vi "Log Writer.vi"(8 "error in (no error)":errorcluster) -> (0 "error out":errorcluster)   [LabVIEW 2026, in "PXI_Common.lvlib"]
uses:
  PXI_Common.lvlib
  Types/Typedef/Log Message Levels.ctl
  Types/Enum/Bench Modules.ctl
  Types/Typedef/Log Message.ctl
panel:
  out "date/time string":string
  in  "Log Table":string[][](table)
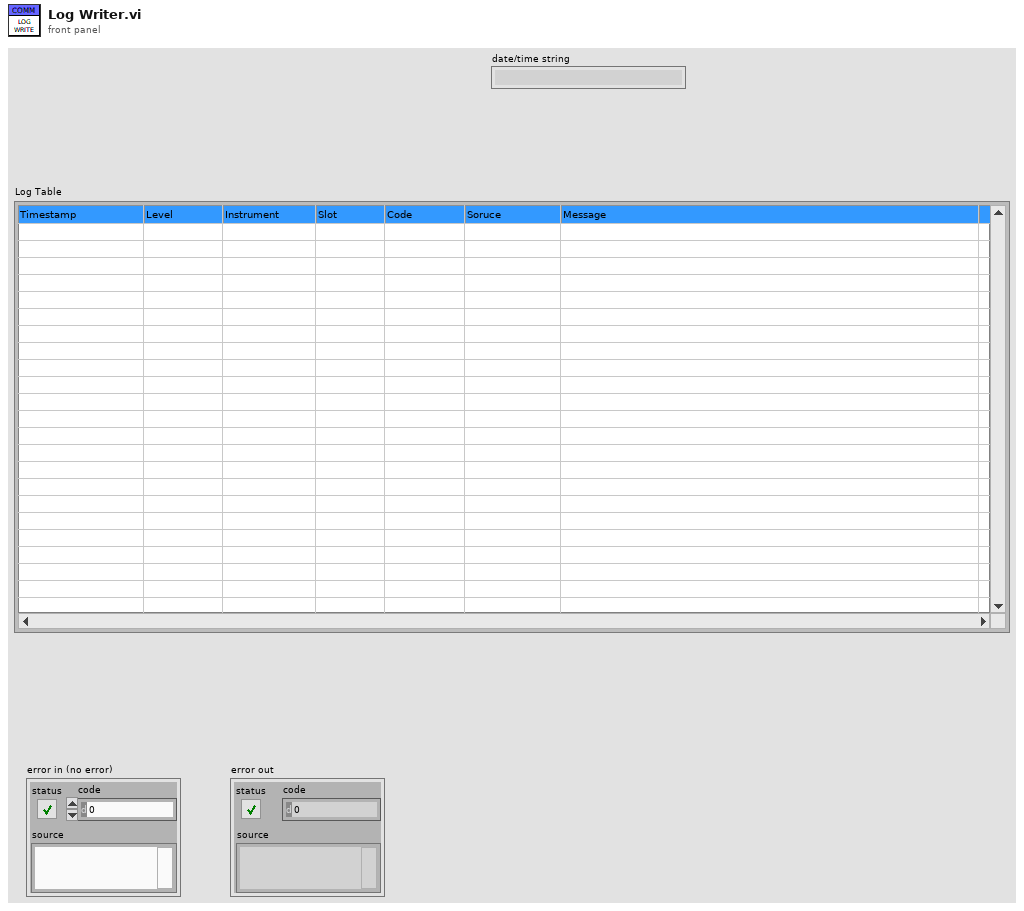
[diagram p1: front panel]
types:
  T1 = typedef "PXI_Common.lvlib/Log Message.ctl" = cluster{"Timestamp":string, "Level":T2, "Instrument":T3, "Slot":string, "Code":i32, "Soruce":string, "Message":string}
  T2 = typedef "PXI_Common.lvlib/Log Message Levels.ctl" = enum16{"DEBUG", "INFO", "WARNING", "ERROR"}
  T3 = typedef "PXI_Common.lvlib/Bench Modules.ctl" = enum16{"Common", "PXI4072", "PXI6259", "PXI6224", "PXI4130", "PXI8431"}
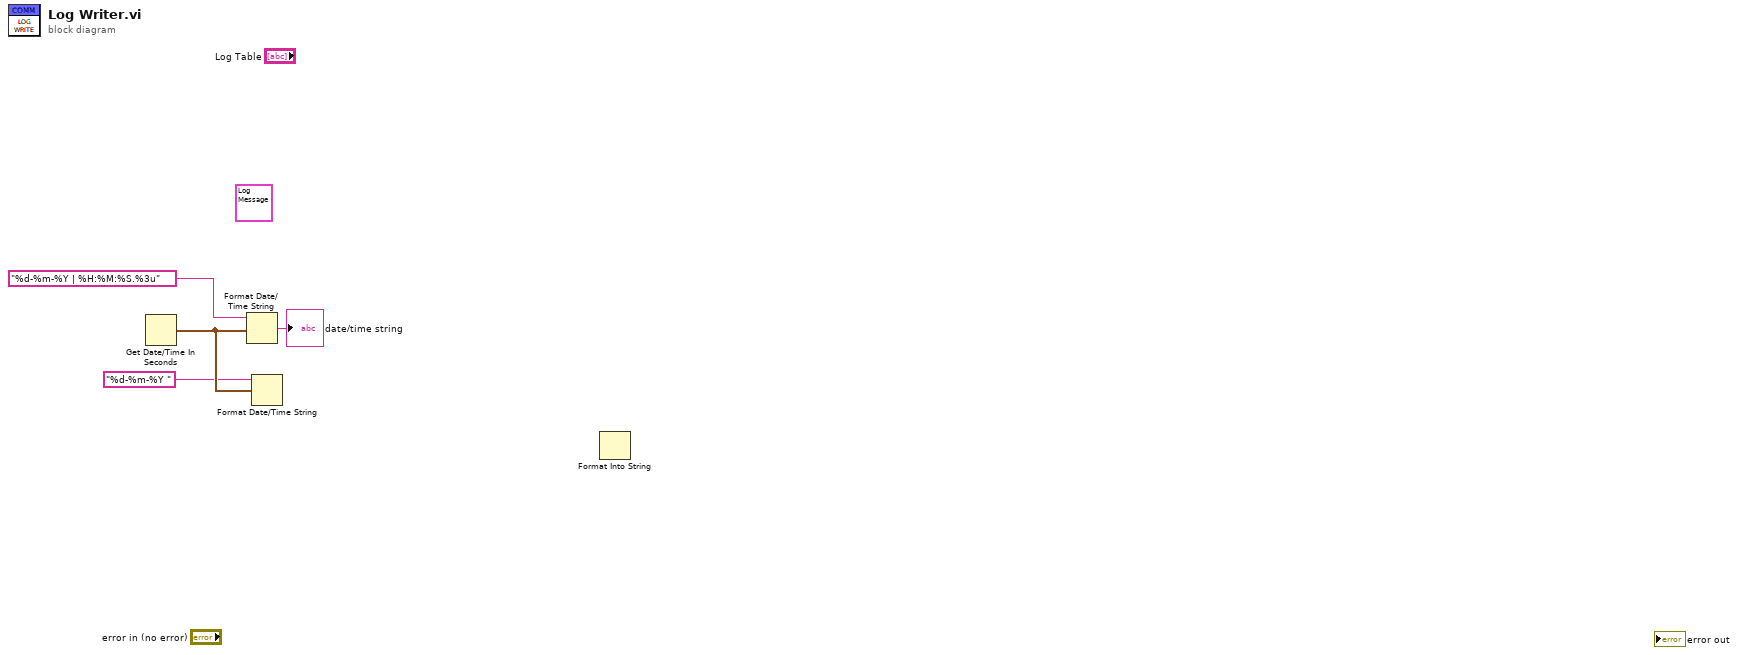
[diagram p0: block diagram]
diagram:
  (unwired) T1 {"Timestamp"="", "Level"=enum."DEBUG", "Instrument"=enum."Common", "Slot"="", "Code"=0, "Soruce"="", "Message"=""} ("Log Message")
  n1 = Get Date/Time In Seconds() -> (seconds since 1Jan1904=w2:timestamp)
  n2 = Format Date/Time String(time format string (%c)="%d-%m-%Y | %H:%M:%S.%3u", seconds (now)=w2) -> (date/time string=→"date/time string":string)  [unwired: 1 in]
  n3 = Format Date/Time String(time format string (%c)="%d-%m-%Y ", seconds (now)=w2) -> ()  [unwired: 1 in, 1 out]
  n4 = Format Into String() -> ()  [unwired: 4 in, 2 out]
